vi "Update Map - Force Move.vi"(8 "Action":cluster{"Action":T1, "Direction":T2}, 9 "Column":i32, 10 "Row":i32, 11 "map dvr in":refnum<data-value>) -> (1 "Selected Direction":T2, 2 "Selected Action":T1, 3 "map dvr out":refnum<data-value>)   [LabVIEW 2015, in "DS Square.lvlib"]
uses:
  DS Square.lvlib
  Common/Position.ctl
  Common/Common.lvlib
  Square State.ctl
  Square Status.ctl
  Type Defs/Action Enum.ctl
  Type Defs/SB Type Defs.lvlib
  Type Defs/Direction Enum.ctl
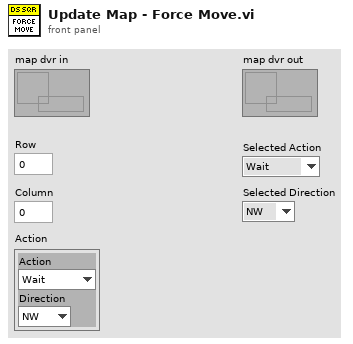
[diagram p1: front panel]
types:
  T1 = typedef "SB Type Defs.lvlib/Action Enum.ctl" = enum16{"Wait", "Move", "Attack", "Replicate"}
  T2 = typedef "SB Type Defs.lvlib/Direction Enum.ctl" = enum16{"NW", "N", "NE", "E", "SE", "S", "SW", "W"}
  T3 = typedef "Common.lvlib/Position.ctl" = cluster{"Column":i32, "Row":i32}
  T4 = typedef "DS Square.lvlib/Square State.ctl" = enum16{"Unknown", "Empty", "Occupied - Active", "Occupied - Cool Down", "Attacked", "Enemy", "Enemy Wall"}
  T5 = typedef "DS Square.lvlib/Square Status.ctl" = cluster{"square state":T4, "probability":dbl, "last update":i32}
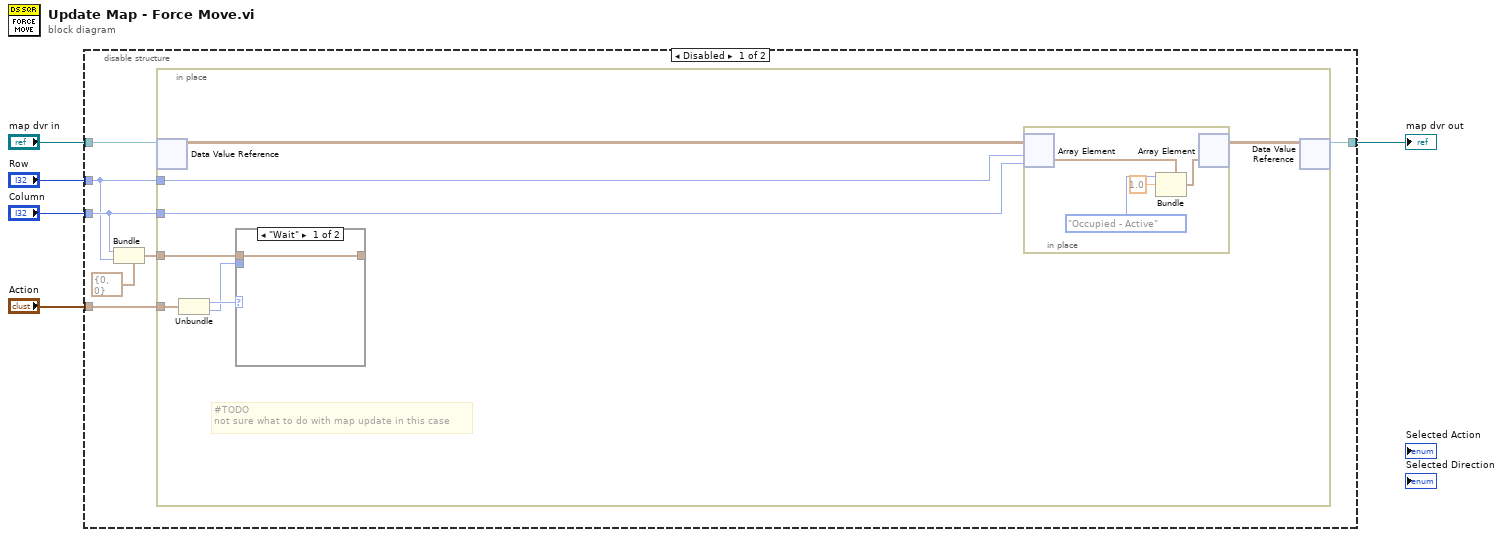
[diagram p0: block diagram]
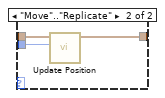
[diagram p2: hidden frame]
diagram:
  n1 = disable-structure shown="Disabled" {
    disable-tunnel: "map dvr in" -> [w12 w29]
    disable-tunnel: [w11 w29] -> w4
    disable-tunnel: "Column" -> [w9 _]
    disable-tunnel: "Row" -> [w8 _]
    disable-tunnel: "Action" -> [w6 _]
    frame Disabled {
      n2 = Bundle(cluster=T3 {"Column"=0, "Row"=0} ("Position in"), "Column"=w9, "Row"=w8) -> (w7:T3)
      n3 = in-place {
        in-place-border: w8 -> [w20]
        in-place-border: w9 -> [w19]
        in-place-border: w7 -> [w16]
        in-place-border: w6 -> [w15]
        # "#TODO\nnot sure what to do with map update in this case"
        n4 = in-place-dvr #1(w12) -> (w17:T5[][])  [unwired: 1 out]
        n5 = Unbundle(w15) -> ("Action"=w14:T1, "Direction"=w13:T2)
        n6 = case shown="\"Wait\"" w14 {
          tunnel: w16 -> [w21 w24]
          tunnel: [w21 w23] -> _
          tunnel: w13 -> [_ w22]
          frame "Wait" {
          }
          frame "Move".."Replicate" {
            n7 = call "Update Position.vi"("Direction"=w22, "Position in"=w24) -> ("Position out"=w23:T3)  [unwired: 9 in]
          }
        }
        n8 = in-place {
          n9 = in-place-array #2(w17, w20, w19) -> (w28:T5)
          n10 = Bundle(cluster=w28, "square state"=Square_State."Occupied - Active", "probability"=1.0) -> (w27:T5)  [unwired: 1 in]
          n11 = in-place-array #2(w27) -> (w18:T5[][])  [unwired: 2 out]
        }
        n12 = in-place-dvr #1(w18) -> (w11:refnum<data-value>)  [unwired: 1 out]
      }
    }
    frame Enabled {
    }
  }
  "map dvr out" <- w4
